vi "OAT IIR Preprocess Filter (N Channels).vi"(0 "scaled signals [EU]":waveform(dbl)[](array[waveform]), 1 "filter type":T3(ring), 2 "reset? (F)":bool, 3 "design method":u16(ring) items=["Butterworth", "Chebyshev", "Inverse Chebyshev", "Elliptic"], 5 "order":i32=2 min=1, 7 "freq specs [Hz]":T2={"low cutoff freq"=100.0, "high cutoff freq"=200.0} {"high cutoff freq" format="%#.2f"; "low cutoff freq" format="%#.4f"}, 9 "ripple specs [dB]":T1={"passband ripple"=0.1, "stopband attenuation"=60.0} {"stopband attenuation" format="%#.2f"; "passband ripple" format="%#.2f"}, 11 "error in (no error)":errorcluster) -> (4 "filtered scaled signals [EU]":waveform(dbl)[](array[waveform]), 15 "error out":errorcluster)   [LabVIEW 2017, in "SoundVib_RefDataProcess.lvlib"]
doc: "Designs an IIR filter and filters the <B>scaled signal [EU]</B>. Each instance of this VI maintains its own state; use the N Waveforms instance of this VI to process an array of channels. Wire data to the <B>scaled signal [EU]</B> input to determine the polymorphic instance to use or manually select the instance."
uses:
  <vilib>/addons/Sound and Vibration/Order Analysis/Referece Data Processing/SoundVib_RefDataProcess.lvlib
  <vilib>/addons/_NISVFA/_Shared subVIs/Common/svc_Check for Waveform Parameter Continuity (no state).vi
  <vilib>/addons/_NISVFA/_Shared subVIs/Common/svc_Get SV Channel Info.vi
  <vilib>/addons/_NISVFA/_Shared subVIs/Common/svc_Engineering Units to Unit Label.vi
  <vilib>/addons/_NISVFA/_Shared subVIs/Common/svc_Unit Label to Engineering Units.vi
  <vilib>/Analysis/NI_AALBase.lvlib
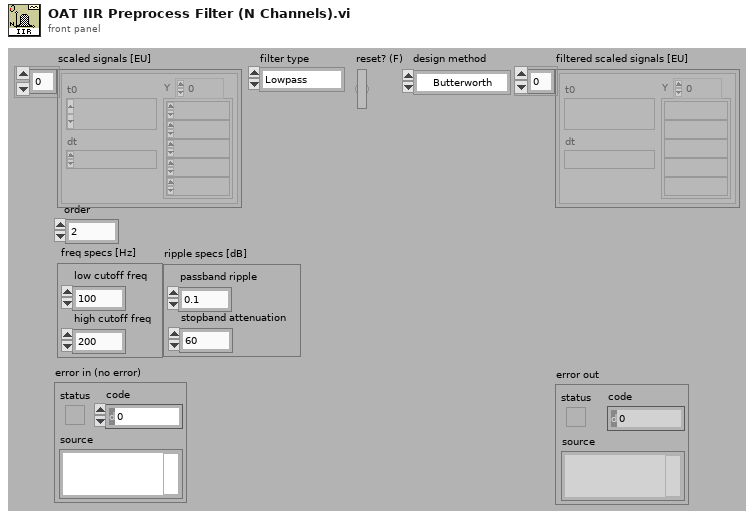
[diagram p1: front panel]
types:
  T1 = cluster{"passband ripple":dbl, "stopband attenuation":dbl}
  T2 = cluster{"low cutoff freq":dbl, "high cutoff freq":dbl}
  T3 = enum32{"Lowpass", "Highpass", "Bandpass", "Bandstop"}
  T4 = cluster{"dt equal":bool, "array length equal":bool, "number channels change":bool}
  T5 = cluster{"dt":bool, "t0 continuity":bool, "array length":bool, "channel info":bool, "name":bool}
  T6 = cluster{"filter structure":enum32{"IIR 2nd Order", "IIR 4th Order"}, "Reverse Coefficients":dbl[], "Forward Coefficients":dbl[]}
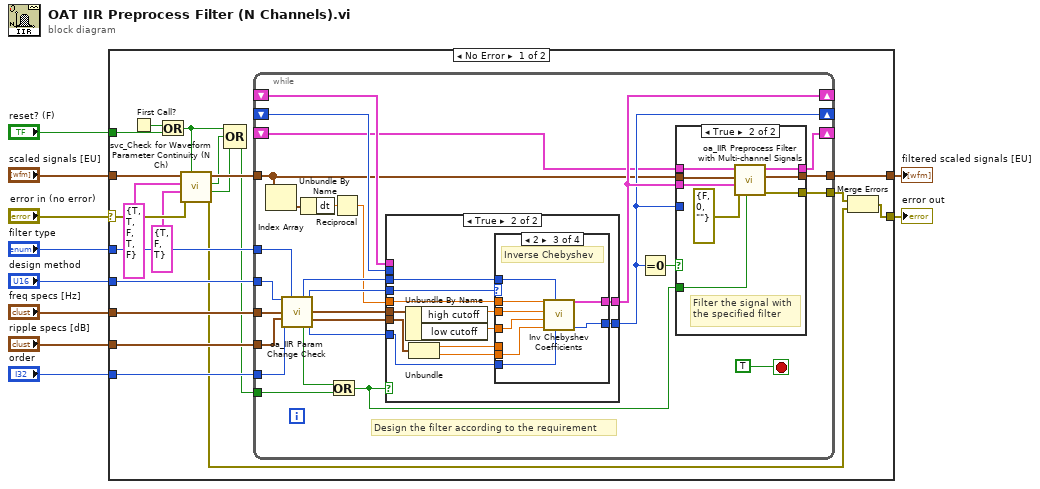
[diagram p0: block diagram]
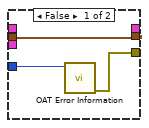
[diagram p2: hidden frame]
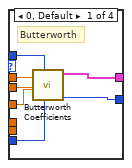
[diagram p4: hidden frame]
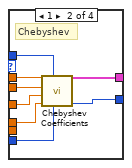
[diagram p5: hidden frame]
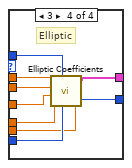
[diagram p6: hidden frame]
diagram:
  n1 = case shown="No Error" "error in (no error)" {
    selector: "error in (no error)" -> [w16 w115]
    tunnel: [w24 w115] -> w10
    tunnel: "scaled signals [EU]" -> [w22 w116]
    tunnel: "design method" -> [w25 _]
    tunnel: "filter type" -> [w27 _]
    tunnel: "order" -> [w26 _]
    tunnel: "freq specs [Hz]" -> [w29 _]
    tunnel: "ripple specs [dB]" -> [w28 _]
    tunnel: [w30 w116] -> w4
    tunnel: "reset? (F)" -> [w15 _]
    frame No Error {
      n2 = First Call?() -> (First Call?: T/F=w23:bool)
      n3 = Or(x=w23, y=w15) -> (x .or. y?=w20:bool)
      n4 = call <vilib>:"svc_Check for Waveform Parameter Continuity (N Ch).vi"("restart averaging (F)"=w20, "error in (no error)"=w16, "checks for multichannel parameters"=T4 {"dt equal"=TRUE, "array length equal"=FALSE, "number channels change"=TRUE}, "checks for channel parameter change"=T5 {"dt"=TRUE, "t0 continuity"=TRUE, "array length"=FALSE, "channel info"=TRUE, "name"=FALSE}, "scaled signal(s)"=w22) -> ("error out"=w13:errorcluster, "multichannel parameter changed"=w18:bool, "waveform parameter changed"=w19:bool, "dup scaled signal(s)"=w21:waveform(dbl)[])  [unwired: 3 out]
      n5 = Compound Arithmetic op=OR(w20, w19, w18) -> (w17:bool)
      n6 = while {
        shift-right: [w44] -> _
        shift-left: _ -> [w36]
        tunnel: w21 -> [w35]
        tunnel: [w49] -> w30
        shift-right: [w41] -> _
        shift-left: _ -> [w47]
        shift-right: [w40] -> _
        shift-left: _ -> [w46]
        tunnel: w29 -> [w45]
        tunnel: w28 -> [w33]
        tunnel: w27 -> [w43]
        tunnel: w26 -> [w42]
        tunnel: [w39] -> w14
        tunnel: w25 -> [w37]
        tunnel: w17 -> [w32]
        stop <- TRUE stop-if-true
        # "Design the filter according to the requirement"
        n7 = Index Array(array=w35) -> (element=w34:waveform(dbl))  [unwired: 1 in]
        n8 = call <vilib>:"oa_IIR Param Change Check.vi"("design method in"=w37, "filter type in"=w43, "freq specs in"=w45, "ripple specs in [dB]"=w33, "order in"=w42) -> ("filter type out"=w57:T3, "design method out"=w56:u16, "freq specs out"=w53:cluster{"low cutoff":dbl, "high cutoff":dbl}, "ripple specs out [dB]"=w52:cluster{"pass band":dbl, "stop band":dbl}, "chang?"=w51:bool, "order out"=w54:i32)  [unwired: 4 in, 1 out]
        n9 = Unbundle By Name(w34) -> ("dt"=w50:dbl)
        n10 = Or(x=w51, y=w32) -> (x .or. y?=w55:bool)
        n11 = Reciprocal(x=w50) -> (1/x=w31:dbl)
        n12 = case shown="True" w55 {
          tunnel: [w69 w82] -> w40
          tunnel: [w70 w81] -> w41
          tunnel: w47 -> [w70 _]
          tunnel: w46 -> [w69 _]
          tunnel: w56 -> [_ w80]
          tunnel: w57 -> [_ w79]
          tunnel: w53 -> [_ w76]
          tunnel: w52 -> [_ w75]
          tunnel: w54 -> [_ w78]
          tunnel: w31 -> [_ w77]
          frame False {
          }
          frame True {
            n13 = Unbundle By Name(w76) -> ("high cutoff"=w74:dbl, "low cutoff"=w73:dbl)
            n14 = Unbundle(w75) -> ("pass band"=w72:dbl, "stop band"=w71:dbl)
            n15 = case shown="2" w80 {
              tunnel: [w89 w97 w105 w114] -> w81
              tunnel: [w88 w96 w104 w113] -> w82
              tunnel: w79 -> [w87 w95 w103 w112]
              tunnel: w78 -> [w83 w90 w98 w107]
              tunnel: w77 -> [w86 w94 w102 w111]
              tunnel: w74 -> [w85 w93 w101 w110]
              tunnel: w73 -> [w84 w92 w100 w109]
              tunnel: w72 -> [_ w91 _ w108]
              tunnel: w71 -> [_ _ w99 w106]
              frame 0, Default {
                # "Butterworth"
                n16 = call <vilib>:"Butterworth Coefficients.vi"("order"=w83, "filter type"=w87, "low cutoff freq: fl"=w84, "high cutoff freq: fh"=w85, "sampling freq: fs"=w86) -> ("error"=w88:i32, "IIR Filter Cluster"=w89:T6)  [unwired: 5 in]
              }
              frame 1 {
                # "Chebyshev"
                n17 = call <vilib>:"Chebyshev Coefficients.vi"("order"=w90, "filter type"=w95, "ripple(dB)"=w91, "low cutoff freq: fl"=w92, "high cutoff freq: fh"=w93, "sampling freq: fs"=w94) -> ("error"=w96:i32, "IIR Filter Cluster"=w97:T6)  [unwired: 4 in]
              }
              frame 2 {
                # "Inverse Chebyshev"
                n18 = call <vilib>:"Inv Chebyshev Coefficients.vi"("order"=w98, "filter type"=w103, "attenuation (dB)"=w99, "low cutoff freq: fl"=w100, "high cutoff freq: fh"=w101, "sampling freq: fs"=w102) -> ("error"=w104:i32, "IIR Filter Cluster"=w105:T6)  [unwired: 4 in]
              }
              frame 3 {
                # "Elliptic"
                n19 = call <vilib>:"Elliptic Coefficients.vi"("stopband attenuation (dB)"=w106, "order"=w107, "filter type"=w112, "passband ripple (dB)"=w108, "low cutoff freq: fl"=w109, "high cutoff freq: fh"=w110, "sampling freq: fs"=w111) -> ("error"=w113:i32, "IIR Filter Cluster"=w114:T6)  [unwired: 3 in]
              }
            }
          }
        }
        n20 = Equal To 0?(x=w40) -> (x = 0?=w38:bool)
        n21 = case shown="True" w38 {
          tunnel: w35 -> [w60 w67]
          tunnel: [w60 w62] -> w49
          tunnel: [_ w61] -> w44
          tunnel: w55 -> [_ w64]
          tunnel: w41 -> [_ w66]
          tunnel: w40 -> [w59 _]
          tunnel: [w58 w63] -> w39
          tunnel: w36 -> [_ w68]
          frame False {
            n22 = call <vilib>:"OAT Error Information.vi"("error code"=w59) -> ("error out"=w58:errorcluster)  [unwired: 6 in]
          }
          frame True {
            # "Filter the signal with\nthe specified filter"
            n23 = call <vilib>:"oa_IIR Preprocess Filter with Multi-channel Signals.vi"("reset"=w64, "error in (no error)"=errorcluster {"status"=FALSE, "code"=0, "source"=""} ("error out"), "IIR Filter Cluster"=w66, "signals in"=w67, "filter history in"=w68) -> ("error out"=w63:errorcluster, "signals out"=w62:waveform(dbl)[], "filter history out"=w61:cluster{"shift register type":dbl[]}[])  [unwired: 4 in]
          }
        }
      }
      n24 = Merge Errors(w14, w13) -> (w24:errorcluster)
    }
    frame Error {
    }
  }
  "error out" <- w10
  "filtered scaled signals [EU]" <- w4
